vi "拆分运算.vi"(3 "公式":string) -> (0 "符号":string[](array[string]), 1 "元素":string[](array[string]))   [LabVIEW 2014]
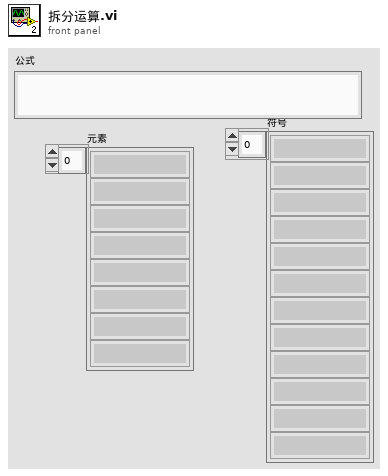
[diagram p1: front panel]
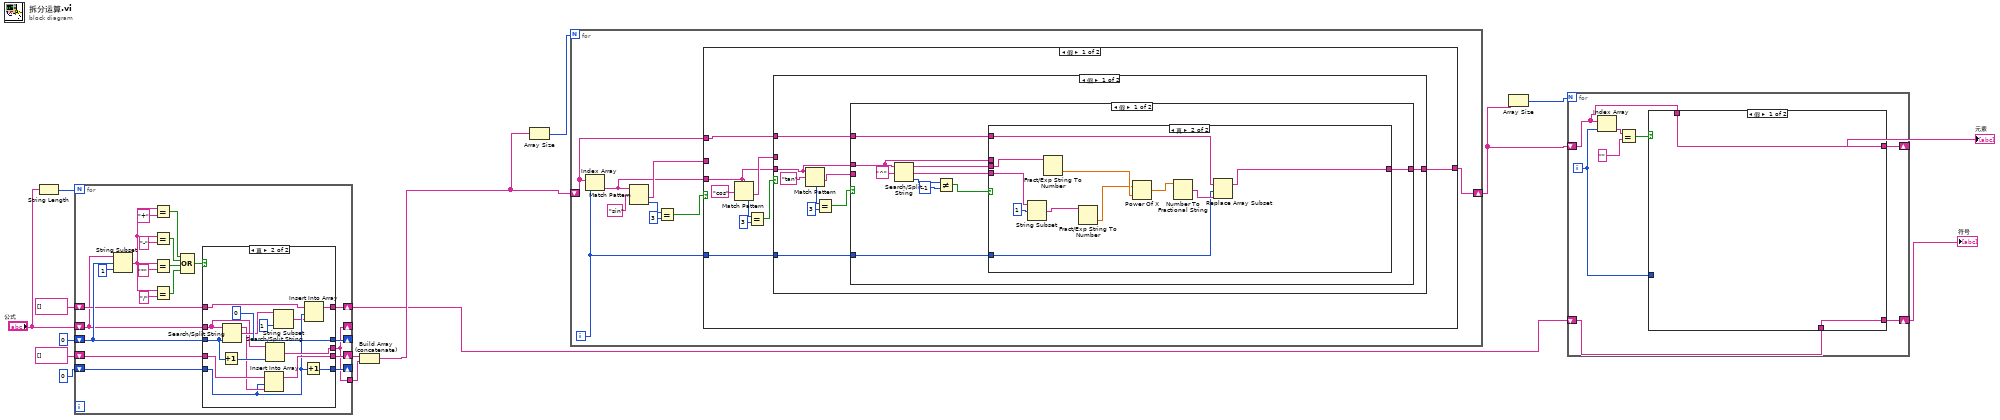
[diagram p0: block diagram]
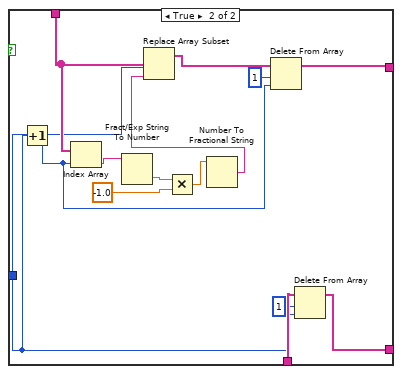
[diagram p2: hidden frame]
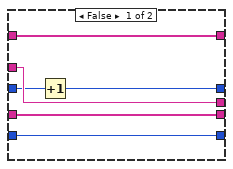
[diagram p3: hidden frame]
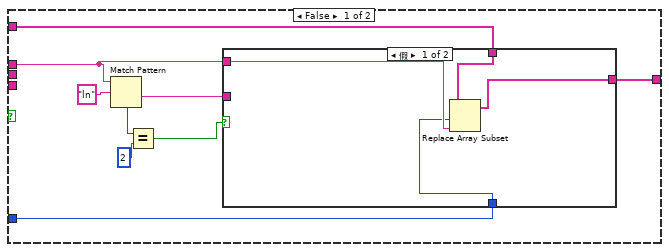
[diagram p4: hidden frame]
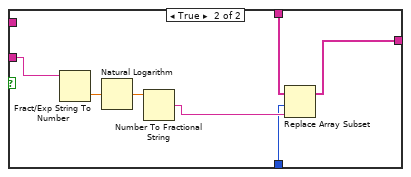
[diagram p5: hidden frame]
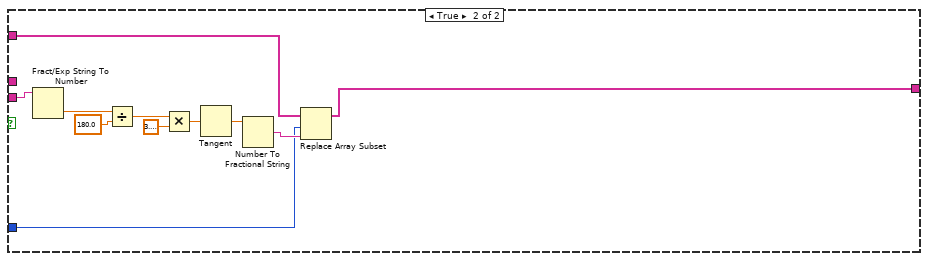
[diagram p6: hidden frame]
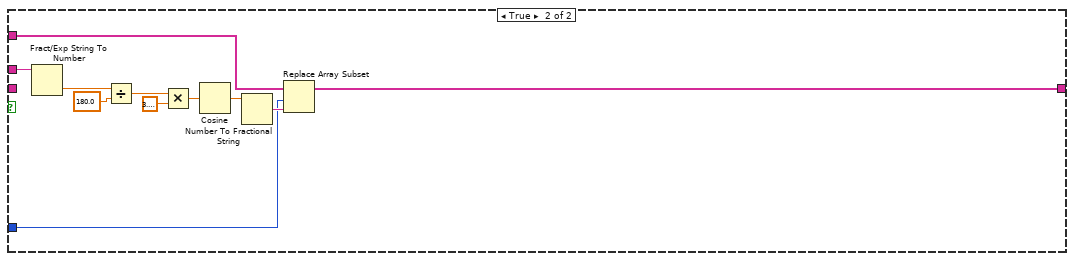
[diagram p7: hidden frame]
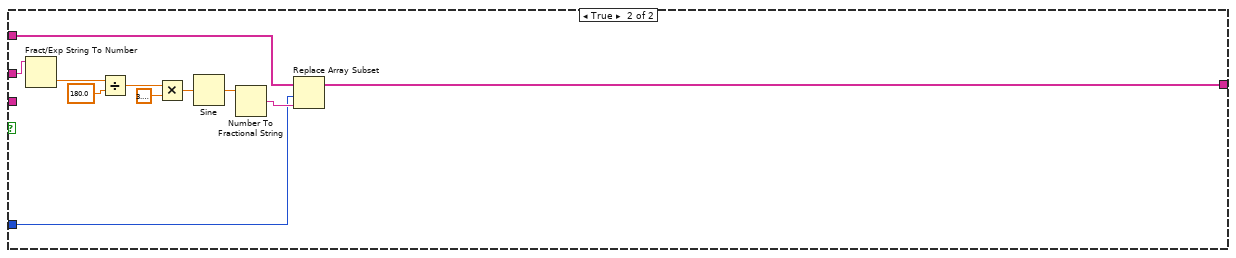
[diagram p8: hidden frame]
diagram:
  n1 = String Length(string="公式") -> (length=w14:i32)
  n2 = for {
    N: w14 -> [_]
    shift-right: [w17] -> _
    shift-left: "公式" -> [w16]
    shift-right: [w24] -> _
    shift-left: 0 -> [w25]
    shift-right: [w23] -> w11
    shift-left: string[] [] -> [w22]
    shift-right: [w20] -> _
    shift-left: 0 -> [w21]
    shift-right: [w18] -> w2
    shift-left: string[] [] -> [w19]
    tunnel: [w17] -> w12
    n3 = String Subset(string=w16, offset (0)=w25, length (rest)=1) -> (substring=w31:string)
    n4 = Equal?(x=w31, y="+") -> (x = y?=w30:bool)
    n5 = Equal?(x=w31, y="-") -> (x = y?=w29:bool)
    n6 = Equal?(x=w31, y="*") -> (x = y?=w28:bool)
    n7 = Equal?(x=w31, y="/") -> (x = y?=w27:bool)
    n8 = Compound Arithmetic op=OR(w30, w29, w28, w27) -> (w26:bool)
    n9 = case shown="真" w26 {
      tunnel: [w42 w52] -> w17
      tunnel: w16 -> [w42 w54]
      tunnel: w25 -> [w41 w51]
      tunnel: [w40 0] -> w24
      tunnel: [w39 w50] -> w23
      tunnel: w22 -> [w39 w49]
      tunnel: w21 -> [w37 w45]
      tunnel: [w37 w47] -> w20
      tunnel: w19 -> [w38 w46]
      tunnel: [w38 w44] -> w18
      frame False {
        n10 = Increment(x=w41) -> (x+1=w40:i32)
      }
      frame True {
        n11 = Increment(x=w51) -> (x+1=w53:i32)
        n12 = Search/Split String(string=w54, offset (0)=w51) -> (substring before match=w48:string, match + rest of string=w56:string)  [unwired: 1 in, 1 out]
        n13 = Insert Into Array(array=w49, index=w45, new element=w48) -> (w50:string[])
        n14 = Search/Split String(string=w54, offset (0)=w53) -> (match + rest of string=w52:string)  [unwired: 1 in, 2 out]
        n15 = String Subset(string=w56, length (rest)=1 ("长度（剩余）")) -> (substring=w43:string)  [unwired: 1 in]
        n16 = Increment(x=w45) -> (x+1=w47:i32)
        n17 = Insert Into Array(array=w46, index=w45, new element=w43) -> (w44:string[])
      }
    }
  }
  n18 = Build Array (concatenate)(w11, w12) -> (w6:string[])
  n19 = Array Size(array=w6) -> (size(s)=w15:i32)
  n20 = for {
    N: w15 -> [_]
    shift-right: [w58] -> w4
    shift-left: w6 -> [w61]
    i -> [w60]
    n21 = Index Array(array=w61, index=w60) -> (element=w59:string)
    n22 = Match Pattern(string=w59, regular expression="sin" ("正则表达式")) -> (after substring=w62:string, offset past match=w65:i32)  [unwired: 1 in, 2 out]
    n23 = Equal?(x=w65, y=3) -> (x = y?=w63:bool)
    n24 = case shown="假" w63 {
      tunnel: w62 -> [_ w158]
      tunnel: w61 -> [w70 w151]
      tunnel: w60 -> [w67 w149]
      tunnel: [w69 w148] -> w58
      tunnel: w59 -> [w68 _]
      frame False {
        n25 = Match Pattern(string=w68, regular expression="cos" ("正则表达式")) -> (after substring=w71:string, offset past match=w74:i32)  [unwired: 1 in, 2 out]
        n26 = Equal?(x=w74, y=3) -> (x = y?=w72:bool)
        n27 = case shown="假" w72 {
          tunnel: w71 -> [_ w142]
          tunnel: w70 -> [w79 w139]
          tunnel: [w77 w138] -> w69
          tunnel: w68 -> [w76 _]
          tunnel: w67 -> [w78 w137]
          frame False {
            n28 = Match Pattern(string=w76, regular expression="tan" ("正则表达式")) -> (after substring=w80:string, offset past match=w83:i32)  [unwired: 1 in, 2 out]
            n29 = Equal?(x=w83, y=3) -> (x = y?=w81:bool)
            n30 = case shown="假" w81 {
              tunnel: w80 -> [_ w129]
              tunnel: w79 -> [w87 w128]
              tunnel: w78 -> [w88 w127]
              tunnel: [w86 w126] -> w77
              tunnel: w76 -> [w85 _]
              frame False {
                n31 = Search/Split String(string=w85, search string/char (-)="^" ("搜索字符串/字符(-)")) -> (substring before match=w90:string, match + rest of string=w89:string, offset of match=w93:i32)  [unwired: 1 in]
                n32 = Not Equal?(x=w93, y=-1) -> (x != y?=w91:bool)
                n33 = case shown="真" w91 {
                  tunnel: w90 -> [_ w118]
                  tunnel: w89 -> [_ w125]
                  tunnel: w88 -> [w98 w121]
                  tunnel: w87 -> [w97 w120]
                  tunnel: [w96 w119] -> w86
                  tunnel: w85 -> [w95 _]
                  frame False {
                    n34 = Match Pattern(string=w95, regular expression="ln" ("正则表达式")) -> (after substring=w99:string, offset past match=w102:i32)  [unwired: 1 in, 2 out]
                    n35 = Equal?(x=w102, y=2) -> (x = y?=w100:bool)
                    n36 = case shown="假" w100 {
                      tunnel: w99 -> [_ w114]
                      tunnel: w98 -> [w106 w110]
                      tunnel: w97 -> [w105 w109]
                      tunnel: [w104 w108] -> w96
                      tunnel: w95 -> [w107 _]
                      frame False {
                        n37 = Replace Array Subset(array=w105, new element=w107, index=w106) -> (w104:string[])
                      }
                      frame True {
                        n38 = Fract/Exp String To Number(string=w114) -> (number=w113:dbl)  [unwired: 3 in, 1 out]
                        n39 = Natural Logarithm(1:w113) -> (0:w112:dbl)
                        n40 = Number To Fractional String(number=w112) -> (F-format string=w111:string)  [unwired: 3 in]
                        n41 = Replace Array Subset(array=w109, new element=w111, index=w110) -> (w108:string[])
                      }
                    }
                  }
                  frame True {
                    n42 = String Subset(string=w125, offset (0)=1 ("偏移量(0)")) -> (substring=w116:string)  [unwired: 1 in]
                    n43 = Fract/Exp String To Number(string=w118) -> (number=w117:dbl)  [unwired: 3 in, 1 out]
                    n44 = Fract/Exp String To Number(string=w116) -> (number=w115:dbl)  [unwired: 3 in, 1 out]
                    n45 = Power Of X(1:w117, 2:w115) -> (0:w123:dbl)
                    n46 = Number To Fractional String(number=w123) -> (F-format string=w122:string)  [unwired: 3 in]
                    n47 = Replace Array Subset(array=w120, new element=w122, index=w121) -> (w119:string[])
                  }
                }
              }
              frame True {
                n48 = Fract/Exp String To Number(string=w129) -> (number=w136:dbl)  [unwired: 3 in, 1 out]
                n49 = Divide(x=w136, y=180.0) -> (x/y=w134:dbl)
                n50 = Multiply(x=w134, y=3.141592653589793) -> (x*y=w132:dbl)
                n51 = Tangent(1:w132) -> (0:w131:dbl)
                n52 = Number To Fractional String(number=w131) -> (F-format string=w130:string)  [unwired: 3 in]
                n53 = Replace Array Subset(array=w128, new element=w130, index=w127) -> (w126:string[])
              }
            }
          }
          frame True {
            n54 = Fract/Exp String To Number(string=w142) -> (number=w147:dbl)  [unwired: 3 in, 1 out]
            n55 = Divide(x=w147, y=180.0) -> (x/y=w145:dbl)
            n56 = Multiply(x=w145, y=3.141592653589793) -> (x*y=w141:dbl)
            n57 = Cosine(x=w141) -> (cos(x)=w140:dbl)
            n58 = Number To Fractional String(number=w140) -> (F-format string=w143:string)  [unwired: 3 in]
            n59 = Replace Array Subset(array=w139, new element=w143, index=w137) -> (w138:string[])
          }
        }
      }
      frame True {
        n60 = Fract/Exp String To Number(string=w158) -> (number=w157:dbl)  [unwired: 3 in, 1 out]
        n61 = Divide(x=w157, y=180.0) -> (x/y=w155:dbl)
        n62 = Multiply(x=w155, y=3.141592653589793) -> (x*y=w153:dbl)
        n63 = Sine(x=w153) -> (sin(x)=w152:dbl)
        n64 = Number To Fractional String(number=w152) -> (F-format string=w150:string)  [unwired: 3 in]
        n65 = Replace Array Subset(array=w151, new element=w150, index=w149) -> (w148:string[])
      }
    }
  }
  n66 = Array Size(array=w4) -> (size(s)=w5:i32)
  n67 = for {
    N: w5 -> [_]
    shift-right: [w161] -> w3
    shift-left: w4 -> [w162]
    shift-right: [w159] -> w1
    shift-left: w2 -> [w160]
    i -> [w163]
    n68 = Index Array(array=w162, index=w163) -> (element=w165:string)
    n69 = Equal?(x=w165, y="") -> (x = y?=w166:bool)
    n70 = case shown="假" w166 {
      tunnel: w163 -> [_ w170]
      tunnel: w162 -> [w168 w178]
      tunnel: [w168 w173] -> w161
      tunnel: w160 -> [w167 w172]
      tunnel: [w167 w169] -> w159
      frame False {
      }
      frame True {
        n71 = Increment(x=w170) -> (x+1=w174:i32)
        n72 = Index Array(array=w178, index=w174) -> (element=w177:string)
        n73 = Fract/Exp String To Number(string=w177) -> (number=w182:dbl)  [unwired: 3 in, 1 out]
        n74 = Multiply(x=w182, y=-1.0) -> (x*y=w180:dbl)
        n75 = Number To Fractional String(number=w180) -> (F-format string=w179:string)  [unwired: 3 in]
        n76 = Replace Array Subset(array=w178, new element=w179, index=w170) -> (w176:string[])
        n77 = Delete From Array(array=w176, length=1 ("长度"), index=w174) -> (array with subset deleted=w173:string[])  [unwired: 1 out]
        n78 = Delete From Array(array=w172, length=1 ("长度"), index=w170) -> (array with subset deleted=w169:string[])  [unwired: 1 out]
      }
    }
  }
  "元素" <- w3
  "符号" <- w1
